vi "notifyError.vi"(7 "error in (no error)":errorcluster, 10 "data passing":T1) -> (0 "error out":errorcluster)   [LabVIEW 2016]
uses:
  data.ctl
  device/device.ctl
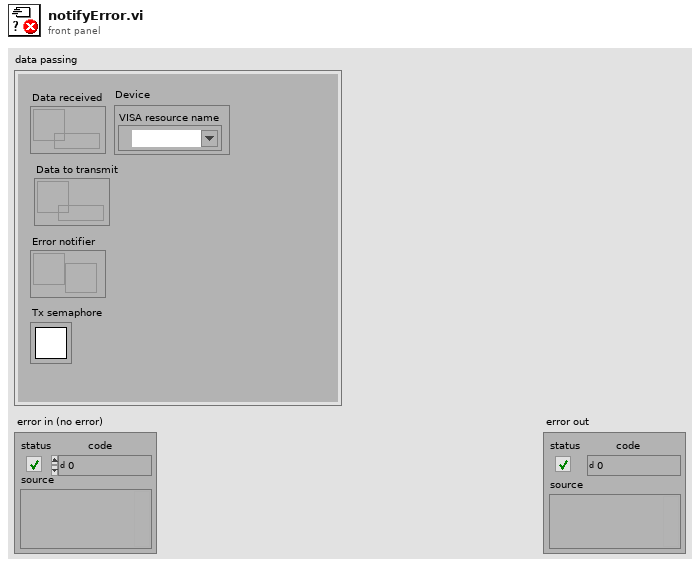
[diagram p1: front panel]
types:
  T1 = typedef "data.ctl" = cluster{"Data received":refnum<queue>, "Data to transmit":refnum<queue>, "Error notifier":refnum<notifier>, "Tx semaphore":T2, "Device":T3}
  T2 = typedef "Semaphore RefNum" = refnum<k1>
  T3 = typedef "device.ctl" = cluster{"VISA resource name":refnum<visa-resource-name>}
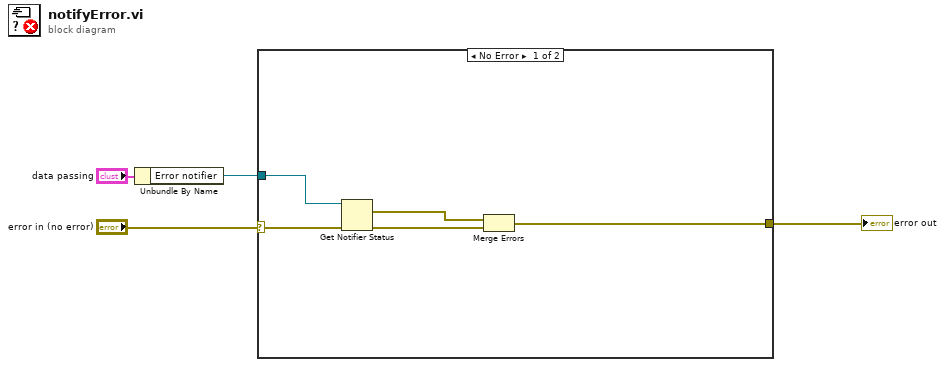
[diagram p0: block diagram]
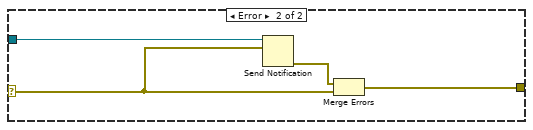
[diagram p2: hidden frame]
diagram:
  n1 = Unbundle By Name("data passing") -> ("Error notifier"=w2:refnum<notifier>)
  n2 = case shown="No Error" "error in (no error)" {
    selector: "error in (no error)" -> [w8 w10]
    tunnel: w2 -> [w9 w13]
    tunnel: [w5 w12] -> w1
    frame No Error {
      n3 = Get Notifier Status(notifier=w9, error in (no error)=w8) -> (current notification=w7:errorcluster, error out=w6:errorcluster)  [unwired: 3 out]
      n4 = Merge Errors(w7, w6) -> (w5:errorcluster)
    }
    frame Error {
      n5 = Send Notification(notification=w10, notifier=w13) -> (error out=w11:errorcluster)  [unwired: 1 in, 1 out]
      n6 = Merge Errors(w11, w10) -> (w12:errorcluster)
    }
  }
  "error out" <- w1
